vi "Test_Resize_ARGB.vi"(8 "error in (no error)":errorcluster, 11 "Test Case In":refnum<class "Image.lvclass">) -> (0 "error out":errorcluster, 3 "Test Case Out":refnum<class "Image.lvclass">)   [LabVIEW 2020, in "g_ar_toolkit.test.lvlib" / "Image.lvclass"]
uses:
  Image.lvclass
  Image.lvclass/Image.ctl
  g_ar_toolkit.image/g_ar_toolkit.image.lvlib
  g_ar_toolkit.image/Image Size (Fixed).ctl
  g_ar_toolkit.image/Interpolation Mode.ctl
  g_ar_toolkit.image/CreateEmptyImageARGB.vi
  g_ar_toolkit.image/ResizeARGB.vi
  4993e8ee-a06a-463a-9684-69129f64d5ce.vi
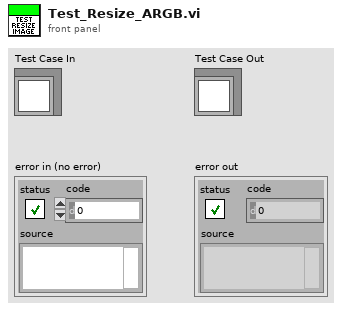
[diagram p1: front panel]
types:
  T1 = typedef "g_ar_toolkit.image.lvlib/Interpolation Mode.ctl" = enum8{"NEAREST", "LINEAR", "CUBIC", "AREA", "LANCZOS", "LINEAR_EXACT", "NEAREST_EXACT", "MAX"}
  T2 = typedef "g_ar_toolkit.image.lvlib/Image Size (Fixed).ctl" = cluster{"Width":u16, "Height":u16}
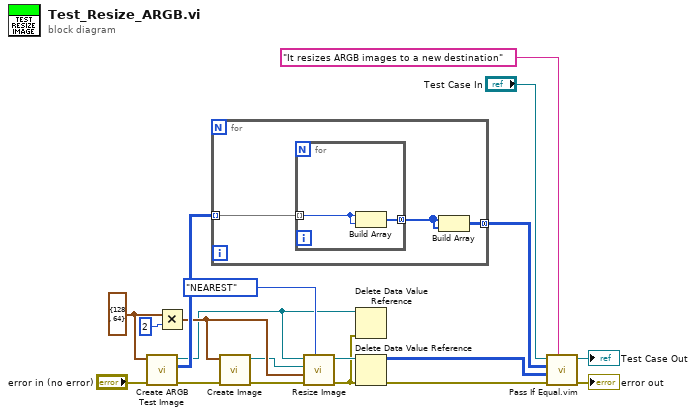
[diagram p0: block diagram]
diagram:
  w11 = T2 {"Width"=128, "Height"=64} ("Preallocated Image Size (Default - 0,0)")
  n1 = call "Create ARGB Test Image.vi"("error in (no error)"="error in (no error)", "Preallocated Image Size"=w11) -> ("error out"=w5:errorcluster, "24-bit pixmap"=w6:u32[][], "Data Value Reference out"=w1:refnum<data-value>)  [unwired: 7 in]
  n2 = Multiply(x=w11, y=u16 2) -> (x*y=w4:T2)
  n3 = for {
    tunnel: w6 -> [w22] mode=indexing
    tunnel: [w20] -> w12 mode=concatenating
    n4 = for {
      tunnel: w22 -> [w24] mode=indexing
      tunnel: [w23] -> w21 mode=concatenating
      n5 = Build Array(w24, w24) -> (w23:u32[])
    }
    n6 = Build Array(w21, w21) -> (w20:u32[][])
  }
  n7 = call-poly "Create Image.vi"("error in (no error)"=w5, "Preallocated Image Size (Default: 0,0)"=w4) -> ("error out"=w9:errorcluster, "New ARGB Image"=w3:refnum<data-value>)  [unwired: 8 in]
  n8 = call-poly "Resize Image.vi"("OpenCV Interpolation Flag (Default: CUBIC)"=Interpolation_Mode."NEAREST" ("OpenCV Interpolation Flag"), "error in (no error)"=w9, "New Image Size"=w4, "ARGB Destination Image"=w3, "ARGB Source Image"=w1) -> ("error out"=w2:errorcluster, "ARGB  Destination Image (duplicate)"=w14:refnum<data-value>)  [unwired: 5 in]
  n9 = Delete Data Value Reference(data value reference=w1, error in=w2) -> ()  [unwired: 2 out]
  n10 = Delete Data Value Reference(data value reference=w14, error in=w2) -> (data value=w8:u32[][], error out=w16:errorcluster)
  n11 = call "Pass If Equal.vim"("Description"="It resizes ARGB images to a new destination", "error in (no error)"=w16, "Actual"=w8, "Expected"=w12, "LUnit Test Case In"="Test Case In") -> ("error out"=→"error out":errorcluster, "LUnit Test Case Out"=→"Test Case Out":refnum<class "Image.lvclass">)  [unwired: 5 in]
